vi "Start Measurement.vi"(8 "error in (no error)":errorcluster, 10 "Launch Measurements Message in":refnum<class "Launch Measurements Message.lvclass">, 11 "TestStand Controller in":refnum<class "Controller API.lvclass">) -> (0 "error out":errorcluster, 3 "TestStand Controller out":refnum<class "Controller API.lvclass">)   [LabVIEW 2016, in "Controller API.lvlib" / "Controller API.lvclass"]
uses:
  <userlib>/Measurement Utility API/Controller API.lvclass
  <userlib>/Common Components/Controller/Messages/Launch Measurements Message/Launch Measurements Message.lvclass
  <userlib>/Measurement Utility API/Messages/Launch Measurement Msg/Launch Measurement and Wait for Result.lvclass
  C:/Program Files (x86)/National Instruments/LabVIEW 2016/user.lib/Common Components/Controller/Messages/Launch Measurements Message/Launch Measurements Message.lvclass
  <userlib>/Measurement Utility API/Messages/Launch Measurement Msg/Launch Measurement and Wait for Result.lvclass/Launch Measurement and Wait for Result.ctl
  <userlib>/Common Components/Controller/Messages/Launch Measurements Message/Launch Measurements Message.lvclass/Launch Measurements Message.ctl
  <userlib>/Measurement Utility API/Controller API.lvclass/Controller API.ctl
  <userlib>/Measurement Utility API/Error Result/Error Report.lvclass
  C:/Program Files (x86)/National Instruments/LabVIEW 2016/user.lib/Common Components/Results/Results.lvclass
  <userlib>/Measurement Utility API/Error Result/Error Report.lvclass/Error Report.ctl
  <userlib>/Common Components/Results/Results.lvclass
  <userlib>/Common Components/Controller/Controller.lvclass
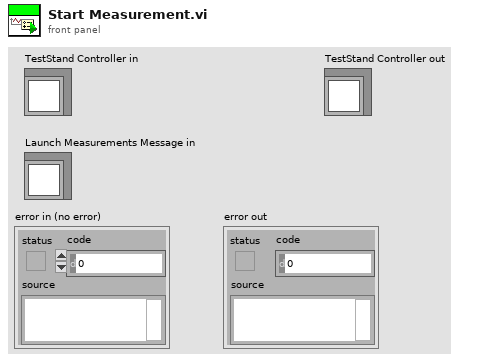
[diagram p1: front panel]
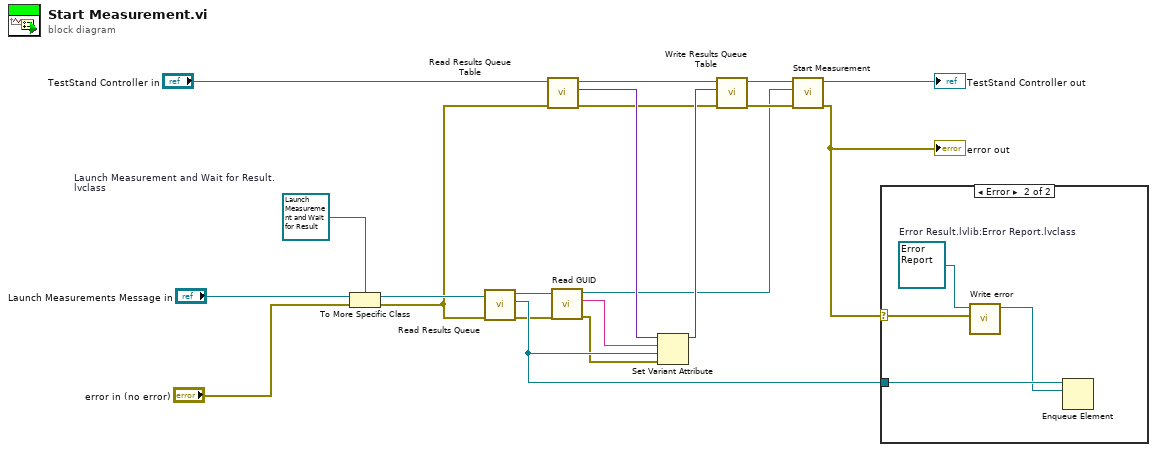
[diagram p0: block diagram]
diagram:
  w18 = refnum<class "Launch Measurement and Wait for Result.lvclass"> refnum  # Launch Measurement and Wait for Result.lvclass
  n1 = To More Specific Class(target class=w18, reference="Launch Measurements Message in", error in="error in (no error)") -> (specific class reference=w6:refnum<class "Launch Measurement and Wait for Result.lvclass">, error out=w5:errorcluster)
  n2 = call <userlib>:"Read Results Queue.vi"("error in (no error)"=w5, "Launch Measurement and Wait for Result in"=w6) -> ("error out"=w4:errorcluster, "Results Queue"=w10:refnum<queue>, "Launch Measurement and Wait for Result out"=w7:refnum<class "Launch Measurement and Wait for Result.lvclass">)  [unwired: 7 in]
  n3 = call <userlib>:"Read Results Queue Table.vi"("error in (no error)"=w5, "TestStand Controller in"="TestStand Controller in") -> ("error out"=w12:errorcluster, "Results Queue Table"=w16:variant, "TestStand Controller out"=w14:refnum<class "Controller API.lvclass">)  [unwired: 7 in]
  n4 = call <userlib>:"Read GUID.vi"("error in (no error)"=w4, "Launch Measurements Message in"=w7) -> ("error out"=w3:errorcluster, "GUID"=w11:string, "Launch Measurements Message out"=w8:refnum<class "Launch Measurement and Wait for Result.lvclass">)  [unwired: 7 in]
  n5 = Set Variant Attribute(Variant=w16, name=w11, value=w10, error in=w3) -> (Variant out=w15:variant)  [unwired: 2 out]
  n6 = call <userlib>:"Write Results Queue Table.vi"("error in (no error)"=w12, "Results Queue Table"=w15, "TestStand Controller in"=w14) -> ("error out"=w9:errorcluster, "TestStand Controller out"=w13:refnum<class "Controller API.lvclass">)  [unwired: 7 in]
  n7 = call-parent "Start Measurement.vi"("error in (no error)"=w9, "Launch Measurements Message in"=w8, "Controller in"=w13) -> ("error out"=w1:errorcluster, "Controller out"=→"TestStand Controller out":refnum<class "Controller API.lvclass">)  [unwired: 7 in]
  "error out" <- w1
  n8 = case shown="Error" w1 {
    selector: w1 -> [_ w21]
    tunnel: w10 -> [_ w23]
    frame No Error {
    }
    frame Error {
      w24 = refnum<class "Error Report.lvclass"> refnum  # Error Result.lvlib:Error Report.lvclass
      n9 = call <userlib>:"Write error.vi"("error"=w21, "Error Report in"=w24) -> ("Error Report out"=w22:refnum<class "Error Report.lvclass">)  [unwired: 8 in, 1 out]
      n10 = Enqueue Element(queue=w23, element=w22) -> ()  [unwired: 2 in, 3 out]
    }
  }
